vi "Exercise 5-2.vi"() -> ()   [LabVIEW 2014]
panel:
  out "Small Cluster":cluster{"Boolean 1":bool, "slide value":dbl}
  out "Modified cluster":T1 {"Slide" scale=0.0..100.0}
  in  "Cluster":T2 {"Slide" scale=0.0..100.0}
  out "Boolean 2":bool
  out "Numeric":dbl
  in  "stop":bool
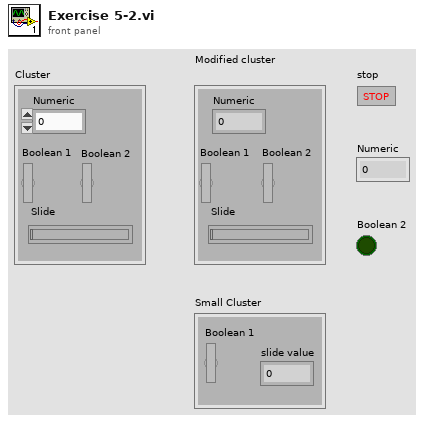
[diagram p1: front panel]
types:
  T1 = cluster{"Numeric":dbl, "Boolean 1":bool, "Boolean 2":bool, "Slide":u8}
  T2 = cluster{"Numeric":dbl, "Boolean 1":bool, "Boolean 2":bool, "Slide":dbl}
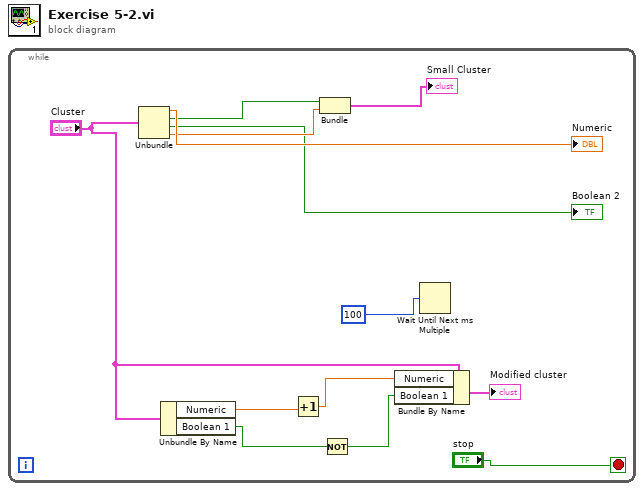
[diagram p0: block diagram]
diagram:
  n1 = while {
    stop <- "stop" stop-if-true
    n2 = Unbundle("Cluster") -> ("Numeric"=→"Numeric":dbl, "Boolean 1"=w11:bool, "Boolean 2"=→"Boolean 2":bool, "Slide"=w12:dbl)
    n3 = Unbundle By Name("Cluster") -> ("Numeric"=w9:dbl, "Boolean 1"=w8:bool)
    n4 = Increment(x=w9) -> (x+1=w7:dbl)
    n5 = Bundle("Boolean 1"=w11, "Slide"=w12) -> (→"Small Cluster":cluster{"Boolean 1":bool, "Slide":dbl})  [unwired: 1 in]
    n6 = Not(x=w8) -> (.not. x?=w4:bool)
    n7 = Bundle By Name(cluster="Cluster", "Numeric"=w7, "Boolean 1"=w4) -> (→"Modified cluster":T2)
    n8 = Wait Until Next ms Multiple(millisecond multiple=100) -> ()  [unwired: 1 out]
  }
